vi "MT_Get.vi"(7 "手动操作(False)":bool, 8 "Error In":errorcluster caption="错误输入", 11 "键盘设备输入":refnum<k1>) -> (0 "Error Out":errorcluster caption="错误输出", 2 "Y轴位置":dbl, 3 "X轴位置":dbl, 4 "Y位置(脉冲)":dbl, 6 "X位置(脉冲)":dbl)   [LabVIEW 2020]
uses:
  <vilib>/Utility/inputDevices.llb/keyboardAcquire.vi
  lib/MT/MT_API.lvlib
panel:
  out "键盘按键显示":string[](array[string])
  out "移动步长(μm)":dbl
  # "获取MT设备位置\n指定是否键盘操作"
  # "手动操作(False)"
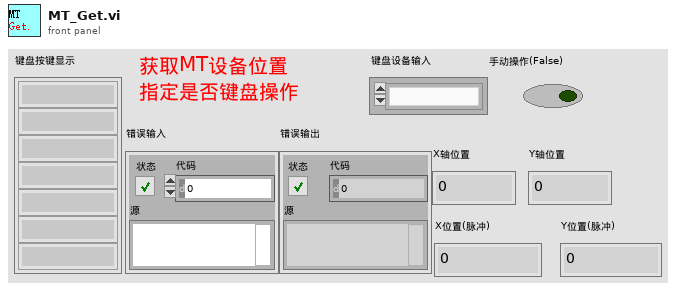
[diagram p1: front panel]
types:
  T1 = enum16{"0", "1", "2", "3", "4", "5", "6", "7", "8", "9", "A", "B", "C", "D", "E", "F", "G", "H", "I", "J", "K", "L", "M", "N", "O", "P", "Q", "R", "S", "T", "U", "V", "W", "X", "Y", "Z", "F1", "F2", "F3", "F4", "F5", "F6", "F7", "F8", "F9", "F10", "F11", "F12", "F13", "F14", "F15", "ADD", "BACK", "BACKSLASH", "CAPITAL", "COMMA", "DECIMAL", "DELETE", "DIVIDE", "DOWN", "END", "EQUALS", "ESCAPE", "GRAVE (`)", "HOME", "INSERT", "LBRACKET", "LCONTROL", "LEFT", "L ALT", "LSHIFT", "LWIN", "MINUS", "MULTIPLY", "NEXT", "NUMLOCK", "NUMPAD_0", "NUMPAD_1", "NUMPAD_2", "NUMPAD_3", "NUMPAD_4", "NUMPAD_5", "NUMPAD_6", "NUMPAD_7", "NUMPAD_8", "NUMPAD_9", "PAUSE", "PERIOD", "PRIOR (PG UP)", "RBRACKET", "RCONTROL", "RETURN", "RIGHT", "R ALT", "RSHIFT", "RWIN", "SCROLL", "SEMICOLON", "SLASH", "SPACE", "SUBTRACT", "TAB", "UP", "ENTER (num pad)", "' (quote)"}[]
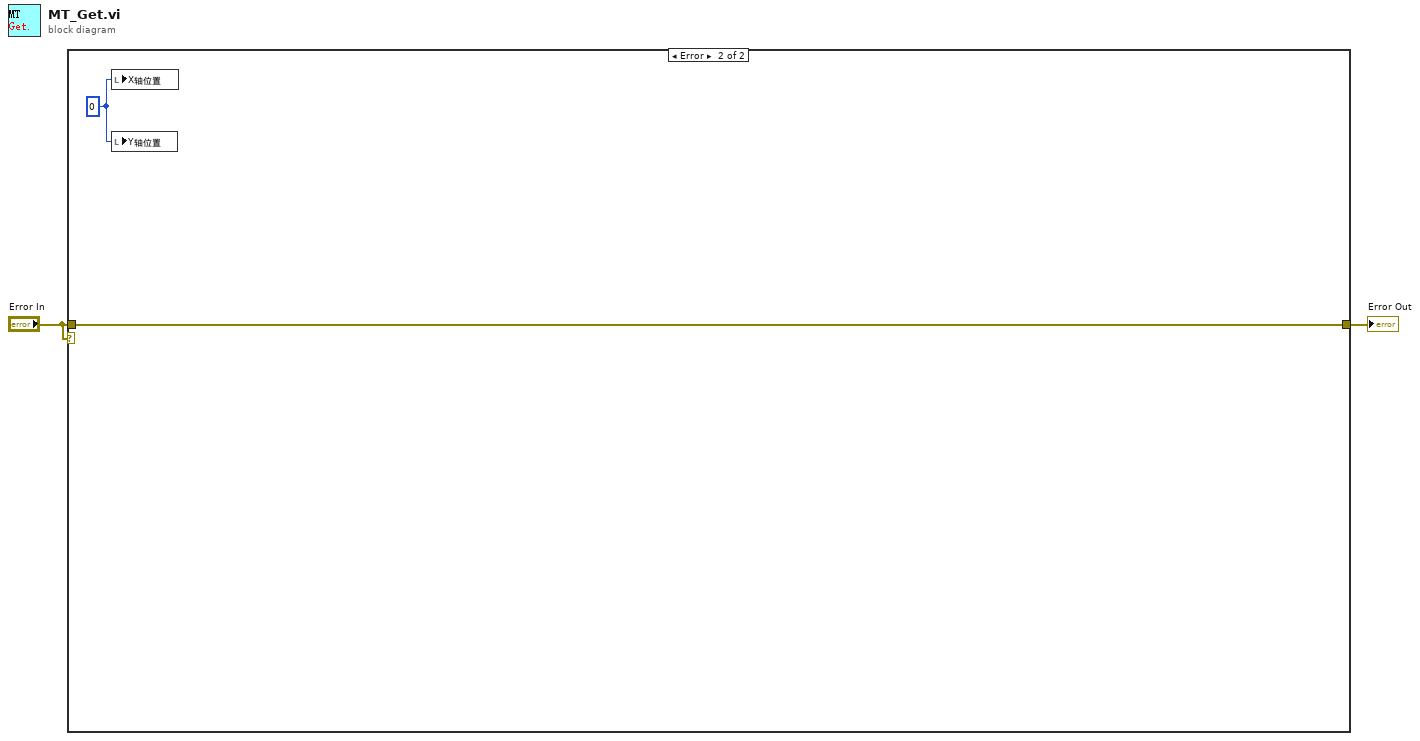
[diagram p0: block diagram]
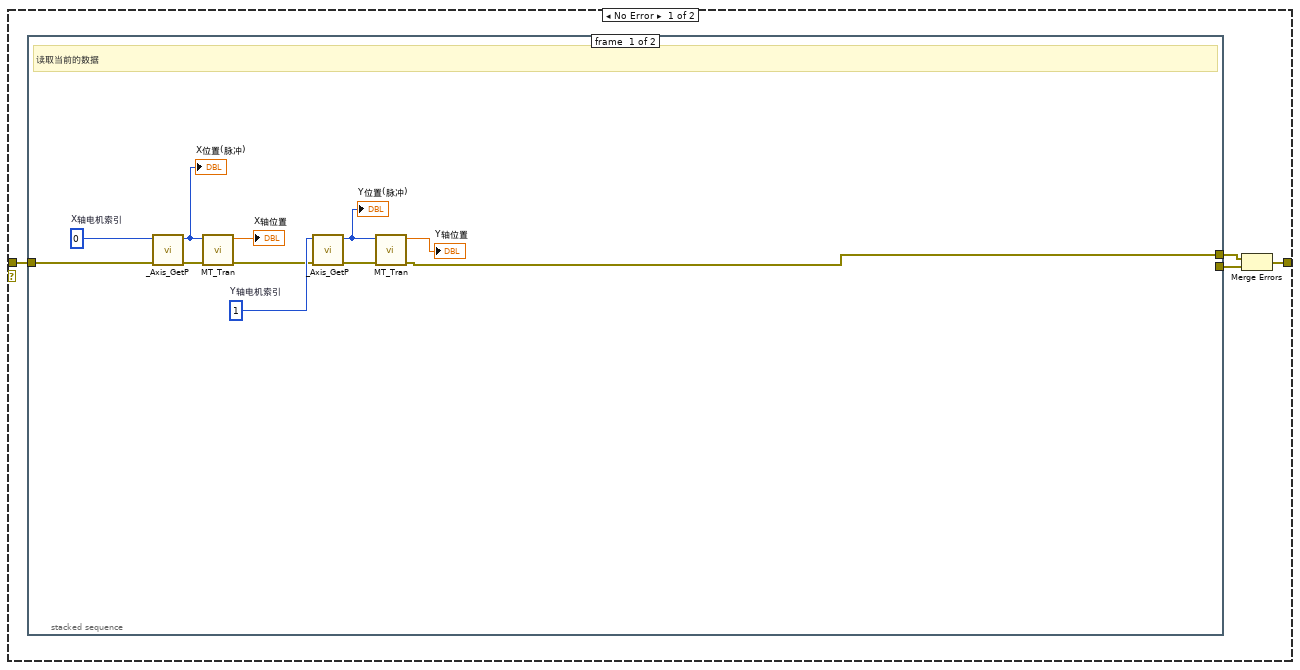
[diagram p2: hidden frame]
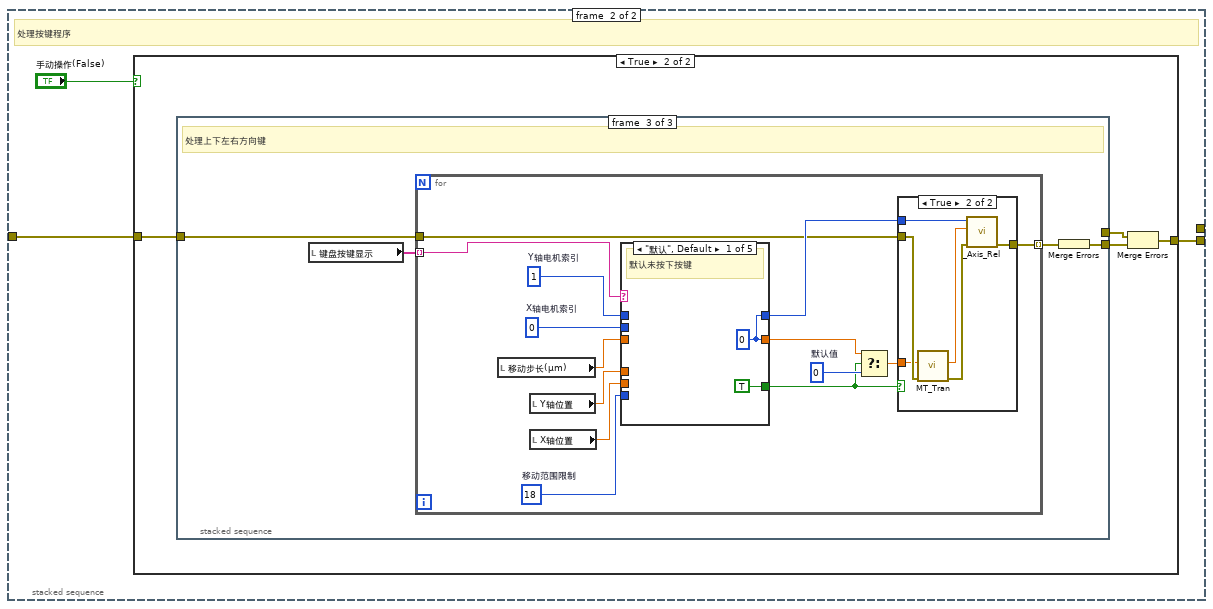
[diagram p3: hidden frame]
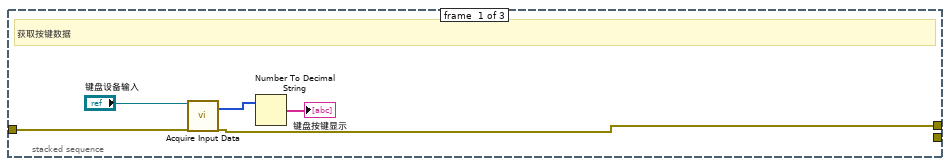
[diagram p5: hidden frame]
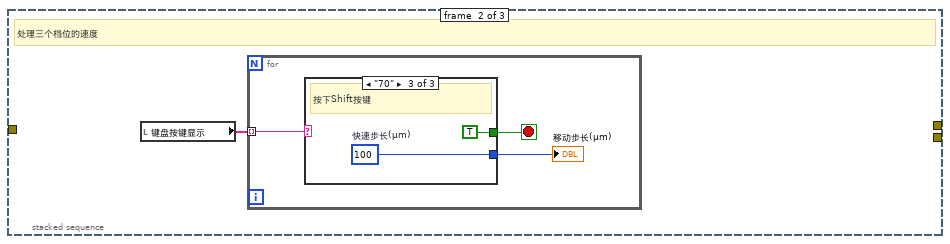
[diagram p6: hidden frame]
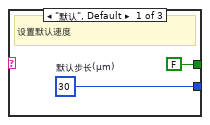
[diagram p7: hidden frame]
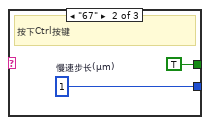
[diagram p8: hidden frame]
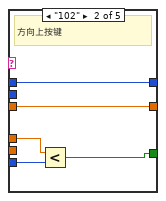
[diagram p10: hidden frame]
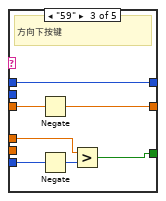
[diagram p11: hidden frame]
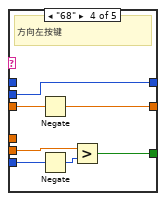
[diagram p12: hidden frame]
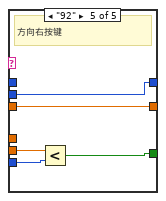
[diagram p13: hidden frame]
diagram:
  n1 = case shown="Error" "Error In" {
    tunnel: [w5 w92] -> w2
    tunnel: "Error In" -> [w6 w92]
    frame No Error {
      n2 = stacked-sequence {
        tunnel: w6 -> [w15 w19]
        tunnel: [w9 _] -> w4
        tunnel: [_ w18] -> w3
        frame #0 {
          w16 = 1  # Y轴电机索引
          w17 = 0  # X轴电机索引
          # "读取当前的数据"
          n3 = call "_Axis_GetP.vi"("Error In"=w15, "轴序号"=w17) -> ("Error Out"=w14:errorcluster, "当前轴对应位置"=w11:i32)  [unwired: 8 in]
          "X位置(脉冲)" <- w11
          n4 = call "MT_Tran.vi"("Error In"=w14, "脉冲个数"=w11) -> ("Error Out"=w13:errorcluster, "位置(mm)"=→"X轴位置":dbl)  [unwired: 6 in, 2 out]
          n5 = call "_Axis_GetP.vi"("Error In"=w13, "轴序号"=w16) -> ("Error Out"=w12:errorcluster, "当前轴对应位置"=w10:i32)  [unwired: 8 in]
          "Y位置(脉冲)" <- w10
          n6 = call "MT_Tran.vi"("Error In"=w12, "脉冲个数"=w10) -> ("Error Out"=w9:errorcluster, "位置(mm)"=→"Y轴位置":dbl)  [unwired: 6 in, 2 out]
        }
        frame #1 {
          # "处理按键程序"
          n7 = case shown="True" "手动操作(False)" {
            tunnel: [w21 w24] -> w18
            tunnel: w19 -> [w21 w22]
            frame False {
            }
            frame True {
              n8 = stacked-sequence {
                tunnel: w22 -> [w28 _ w42]
                tunnel: [w26 _ _] -> w25
                tunnel: [_ _ w41] -> w23
                frame #0 {
                  # "获取按键数据"
                  n9 = call-poly <vilib>:"Acquire Input Data.vi"("device ID"="键盘设备输入", "error in (no error)"=w28) -> ("keys pressed"=w29:T1, "error out"=w26:errorcluster)  [unwired: 15 in, 1 out]
                  n10 = Number To Decimal String(number=w29) -> (decimal integer string=→"键盘按键显示":string[])  [unwired: 1 in]
                }
                frame #1 {
                  # "处理三个档位的速度"
                  n11 = local read "键盘按键显示"() -> (w31:string[])
                  n12 = for {
                    tunnel: w31 -> [w33] mode=indexing
                    stop <- w32 stop-if-true
                    n13 = case "条件结构" shown="\"70\"" w33 {
                      tunnel: [w36 w38 w40] -> w34
                      tunnel: [FALSE TRUE TRUE] -> w32
                      frame "默认", Default {
                        w36 = 30  # 默认步长(μm)
                        # "设置默认速度"
                      }
                      frame "67" {
                        w38 = 1  # 慢速步长(μm)
                        # "按下Ctrl按键"
                      }
                      frame "70" {
                        w40 = 100  # 快速步长(μm)
                        # "按下Shift按键"
                      }
                    }
                    "移动步长(μm)" <- w34
                  }
                }
                frame #2 {
                  # "处理上下左右方向键"
                  n14 = local read "键盘按键显示"() -> (w43:string[])
                  n15 = for {
                    tunnel: w43 -> [w58] mode=indexing
                    tunnel: w42 -> [w49]
                    tunnel: [w48] -> w44 mode=indexing
                    w54 = 0  # 默认值
                    w53 = 1  # Y轴电机索引
                    w51 = 0  # X轴电机索引
                    w56 = 18  # 移动范围限制
                    n16 = local read "移动步长(μm)"() -> (w57:dbl)
                    n17 = local read "Y轴位置"() -> (w55:dbl)
                    n18 = local read "X轴位置"() -> (w52:dbl)
                    n19 = case shown="\"默认\", Default" w58 {
                      tunnel: w57 -> [_ w68 w79 w86 w88]
                      tunnel: [w66 w70 w75 w82 w89] -> w50
                      tunnel: w56 -> [_ w72 w78 w85 w91]
                      tunnel: w55 -> [_ w71 w76 _ _]
                      tunnel: w53 -> [_ w70 w75 _ _]
                      tunnel: w52 -> [_ _ _ w83 w90]
                      tunnel: w51 -> [_ _ _ w82 w89]
                      tunnel: [TRUE w69 w74 w81 w87] -> w45
                      tunnel: [w66 w68 w73 w80 w88] -> w47
                      frame "默认", Default {
                        w66 = 0
                        # "默认未按下按键"
                      }
                      frame "102" {
                        # "方向上按键"
                        n20 = Less?(x=w71, y=w72) -> (x < y?=w69:bool)
                      }
                      frame "59" {
                        # "方向下按键"
                        n21 = Negate(x=w79) -> (-x=w73:dbl)
                        n22 = Negate(x=w78) -> (-x=w77:i32)
                        n23 = Greater?(x=w76, y=w77) -> (0:w74:bool)
                      }
                      frame "68" {
                        # "方向左按键"
                        n24 = Negate(x=w86) -> (-x=w80:dbl)
                        n25 = Negate(x=w85) -> (-x=w84:i32)
                        n26 = Greater?(x=w83, y=w84) -> (0:w81:bool)
                      }
                      frame "92" {
                        # "方向右按键"
                        n27 = Less?(x=w90, y=w91) -> (x < y?=w87:bool)
                      }
                    }
                    n28 = Select(t=w47, s=w45, f=w54) -> (s? t:f=w46:dbl)
                    n29 = case shown="True" w45 {
                      tunnel: w50 -> [_ w64]
                      tunnel: w49 -> [w59 w63]
                      tunnel: w46 -> [_ w62]
                      tunnel: [w59 w60] -> w48
                      frame False {
                      }
                      frame True {
                        n30 = call "MT_Tran.vi"("Error In"=w63, "偏移量(μm)"=w62) -> ("Error Out"=w61:errorcluster, "脉冲个数"=w65:dbl)  [unwired: 6 in, 2 out]
                        n31 = call "_Axis_Rel.vi"("Error In"=w61, "相对位置"=w65, "轴序号"=w64) -> ("Error Out"=w60:errorcluster)  [unwired: 8 in]
                      }
                    }
                  }
                  n32 = Merge Errors(w44) -> (w41:errorcluster)
                }
              }
              n33 = Merge Errors(w25, w23) -> (w24:errorcluster)
            }
          }
        }
      }
      n34 = Merge Errors(w4, w3) -> (w5:errorcluster)
    }
    frame Error {
      w93 = 0
      n35 = local write "X轴位置"(w93) -> ()
      n36 = local write "Y轴位置"(w93) -> ()
    }
  }
  "Error Out" <- w2
